vi "Configure Alternation Trigger (TV).vi"(0 "VISA resource name":refnum<visa-resource-name>, 1 "TV Event (0: All Lines)":u16(ring) items=["All Lines", "Line Number", "Odd Field", "Even Field"], 5 "Trigger Source (0: Source A)":u16(ring) items=["Source A", "Source B"], 7 "TV Trigger Polarity (0: Positive)":u16(ring) items=["Positive", "Negative"], 9 "Signal Format (0: NTSC)":u16(ring) items=["NTSC", "PAL/SECAM"], 11 "error in (no error)":errorcluster, 12 "TV Line Number (1)":i32=1) -> (4 "VISA resource name out":refnum<visa-resource-name>, 15 "error out":errorcluster)   [LabVIEW 2010, in "Agilent DSO1000 Series.lvlib"]
doc: "Configures the TV trigger under alternation trigger mode. You configure the TV trigger source, signal format, the event, and the signal polarity on which to trigger."
uses:
  <instrlib>/Agilent DSO1000 Series/Agilent DSO1000 Series.lvlib
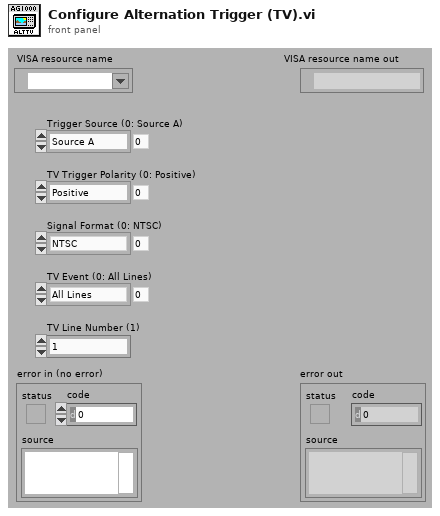
[diagram p1: front panel]
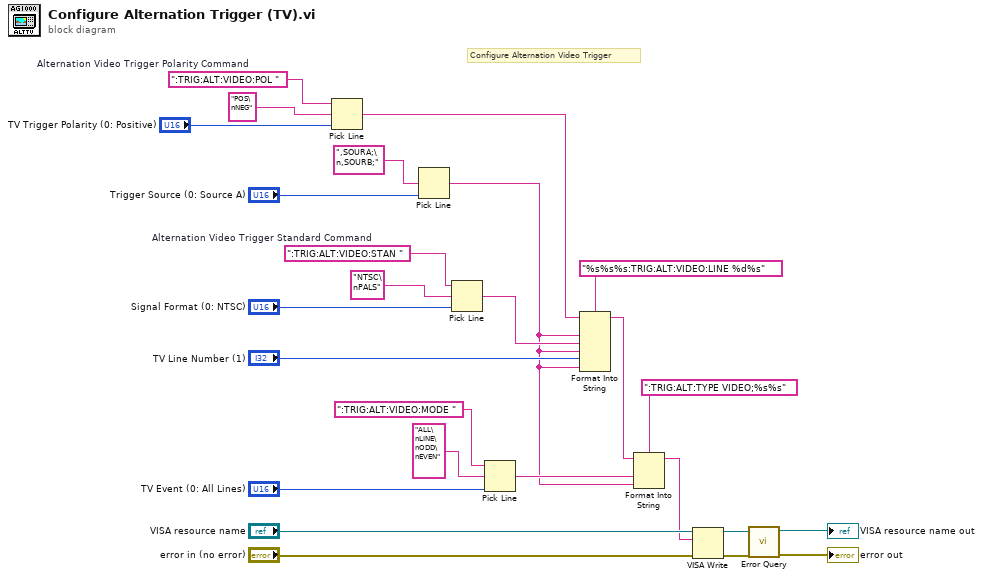
[diagram p0: block diagram]
diagram:
  w17 = ":TRIG:ALT:VIDEO:POL "  # Alternation Video Trigger Polarity Command
  w19 = ":TRIG:ALT:VIDEO:STAN "  # Alternation Video Trigger Standard Command
  # "Configure Alternation Video Trigger"
  n1 = Pick Line(string ("")=w17, multi-line string="POS\nNEG", line index="TV Trigger Polarity (0: Positive)") -> (output string=w5:string)
  n2 = Pick Line(multi-line string=",SOURA;\n,SOURB;", line index="Trigger Source (0: Source A)") -> (output string=w1:string)  [unwired: 1 in]
  n3 = Pick Line(string ("")=w19, multi-line string="NTSC\nPALS", line index="Signal Format (0: NTSC)") -> (output string=w4:string)
  n4 = Pick Line(string ("")=":TRIG:ALT:VIDEO:MODE ", multi-line string="ALL\nLINE\nODD\nEVEN", line index="TV Event (0: All Lines)") -> (output string=w2:string)
  n5 = Format Into String(format string="%s%s%s:TRIG:ALT:VIDEO:LINE %d%s", initial string=w5, w1, w4, w1, "TV Line Number (1)", w1) -> (resulting string=w8:string)  [unwired: 1 in, 1 out]
  n6 = Format Into String(format string=":TRIG:ALT:TYPE VIDEO;%s%s", initial string=w8, w2, w1) -> (resulting string=w6:string)  [unwired: 1 in, 1 out]
  n7 = VISA Write(VISA resource name="VISA resource name", write buffer=w6, error in (no error)="error in (no error)") -> (VISA resource name out=w15:refnum<visa-resource-name>, error out=w14:errorcluster)  [unwired: 1 out]
  n8 = call <instrlib>:"Error Query.vi"("error in (no error)"=w14, "VISA resource name"=w15) -> ("error out"=→"error out":errorcluster, "VISA resource name out"=→"VISA resource name out":refnum<visa-resource-name>)  [unwired: 6 in, 2 out]
